vi "all_path.vi"() -> ()   [LabVIEW 2010]
uses:
  <vilib>/Utility/xml.llb/Read From XML File(string).vi
  <vilib>/Utility/xml.llb/Write to XML File(string).vi
panel:
  out "Array":cluster{dbl[][]}[](array[cluster])
  in  "XML File Path":path
  out "exe?":bool
  out "appended array":path[](array[path])
  out "default = app?":bool
  out "Application Directory":path
  out "data":path
  out "temporary":path
  out "default":path
  out "vi library":path
  out "current":path
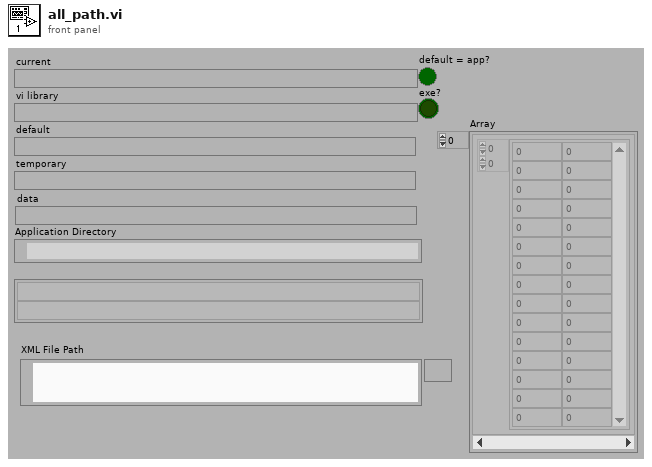
[diagram p1: front panel]
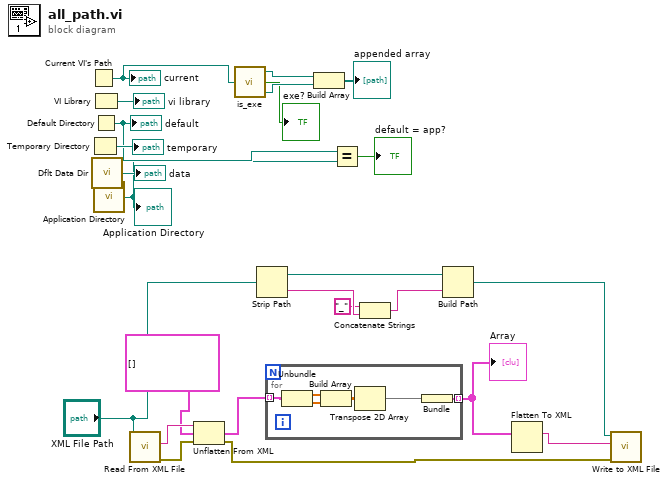
[diagram p0: block diagram]
diagram:
  n1 = Current VI's Path() -> (path=w18:path)
  "current" <- w18
  n2 = Temporary Directory() -> (→"temporary":path)
  n3 = VI Library() -> (path=→"vi library":path)
  n4 = Default Directory() -> (w21:path)
  "default" <- w21
  n5 = call <vilib>:"Dflt Data Dir.vi"() -> ("App:Default Data Directory"=→"data":path)
  n6 = call <vilib>:"Application Directory.vi"() -> ("Application Directory"=w20:path)
  "Application Directory" <- w20
  n7 = call-poly <vilib>:"Read From XML File.vi"("XML File Path"="XML File Path") -> ("error out"=w11:errorcluster, "XML Elements"=w13:string)  [unwired: 8 in, 1 out]
  n8 = Unflatten From XML(xml string=w13, type=cluster{dbl[], dbl[]}[] [], error in (no error)=w11) -> (value=w8:cluster{dbl[], dbl[]}[], error out=w10:errorcluster)
  n9 = call "is_exe.vi"("path"=w18) -> ("actual path"=w16:path, "exe?"=→"exe?":bool, "ini path"=w17:path)  [unwired: 2 in]
  n10 = Strip Path(path="XML File Path") -> (stripped path=w6:path, name=w3:string)
  n11 = for {
    tunnel: w8 -> [w30] mode=indexing
    tunnel: [w26] -> w7 mode=indexing
    n12 = Unbundle(w30) -> (w29:dbl[], w28:dbl[])
    n13 = Build Array(w29, w28) -> (w27:dbl[][])
    n14 = Transpose 2D Array(2D array=w27) -> (transposed array=w25:dbl[][])
    n15 = Bundle(w25) -> (w26:cluster{dbl[][]})  [unwired: 1 in]
  }
  "Array" <- w7
  n16 = Build Array(w17, w16) -> (→"appended array":path[])
  n17 = Equal?(x=w21, y=w20) -> (x = y?=→"default = app?":bool)
  n18 = Concatenate Strings("_" ("string"), w3) -> (w4:string)
  n19 = Build Path(base path=w6, name or relative path=w4) -> (appended path=w1:path)
  n20 = Flatten To XML(anything=w7) -> (xml string=w12:string)
  n21 = call-poly <vilib>:"Write to XML File.vi"("error in (no error)"=w10, "XML Input"=w12, "XML File Path"=w1) -> ()  [unwired: 6 in, 3 out]
